vi "Internet_Checker(SubVI).vi"(2 "error in (no error)":errorcluster) -> (0 "error out":errorcluster, 1 "status":bool)   [LabVIEW 2020]
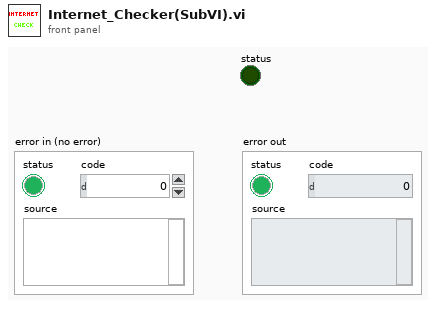
[diagram p1: front panel]
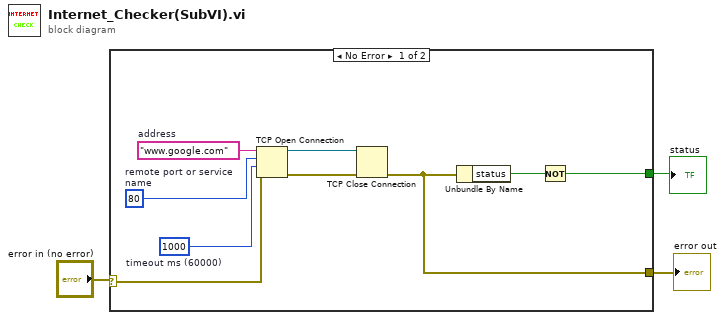
[diagram p0: block diagram]
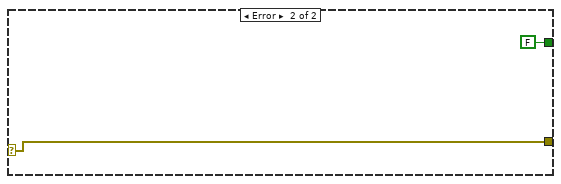
[diagram p2: hidden frame]
diagram:
  n1 = case shown="No Error" "error in (no error)" {
    selector: "error in (no error)" -> [w6 w14]
    tunnel: [w5 w14] -> w2
    tunnel: [w4 FALSE] -> w3
    frame No Error {
      w8 = u16 80  # remote port or service name
      w9 = 1000  # timeout ms (60000)
      w10 = "www.google.com"  # address
      n2 = TCP Open Connection(address=w10, remote port or service name=w8, timeout ms (60000)=w9, error in (no error)=w6) -> (connection ID=w12:refnum<k5>, error out=w11:errorcluster)  [unwired: 1 in]
      n3 = TCP Close Connection(connection ID=w12, error in (no error)=w11) -> (error out=w5:errorcluster)  [unwired: 1 in, 1 out]
      n4 = Unbundle By Name "Unbundle By Name"(w5) -> ("status"=w7:bool)
      n5 = Not(x=w7) -> (.not. x?=w4:bool)
    }
    frame Error {
    }
  }
  "error out" <- w2
  "status" <- w3
